vi "ma_SML Averaged Frequency Response.vi"(6 "reset averaging?":bool, 7 "averaging parameters":T1={"averaging type"=enum."no averaging", "averaging settings"={"weighting type"=enum."linear", "weighting settings"={"size"=10.0, "linear weighting mode"=enum."moving average"}}}, 8 "error in (no error)":errorcluster, 9 "spectral info in":T3 {"window" items=["Rectangle"=0, "Hanning"=1, "Hamming"=2, "Blackman-Harris"=3, "Exact Blackman"=4, "Blackman"=5, "Flat Top"=6, "4 Term B-Harris "=7, "7 Term B-Harris"=8, "Low Sidelobe"=9, "Blackman Nuttall"=11, "Triangle"=30, "Bartlett-Hanning"=31, "Bohman"=32, "Parzen"=33, "Welch"=34, "Kaiser"=60, "Dolph-Chebyshev"=61, "Gaussian"=62]}, 10 "FFTspectrum 2":T4 {"spectrum" format="%.2f"; "df" format="%.2f"; "f0" format="%.2f"}, 11 "FFTspectrum 1":T4 {"spectrum" format="%.2f"; "df" format="%.2f"; "f0" format="%.2f"}) -> (0 "error out":errorcluster, 1 "data ready?":bool, 2 "spectral info out":T3 {"window" items=["Rectangle"=0, "Hanning"=1, "Hamming"=2, "Blackman-Harris"=3, "Exact Blackman"=4, "Blackman"=5, "Flat Top"=6, "4 Term B-Harris "=7, "7 Term B-Harris"=8, "Low Sidelobe"=9, "Blackman Nuttall"=11, "Triangle"=30, "Bartlett-Hanning"=31, "Bohman"=32, "Parzen"=33, "Welch"=34, "Kaiser"=60, "Dolph-Chebyshev"=61, "Gaussian"=62]}, 3 "averaged frequency response":T4 {"spectrum" format="%.2f"; "df" format="%.2f"; "f0" format="%.2f"}, 4 "averages sofar":dbl)   [LabVIEW 2020, in "NI_MAPro.lvlib"]
uses:
  NI_MAPro.lvlib
  ma_sml_Spectrum Cluster (complex).ctl
  ma_sml_Spectral Info.ctl
  ma_sml_Averaging Parameters.ctl
  ma_sml_Averaging Settings.ctl
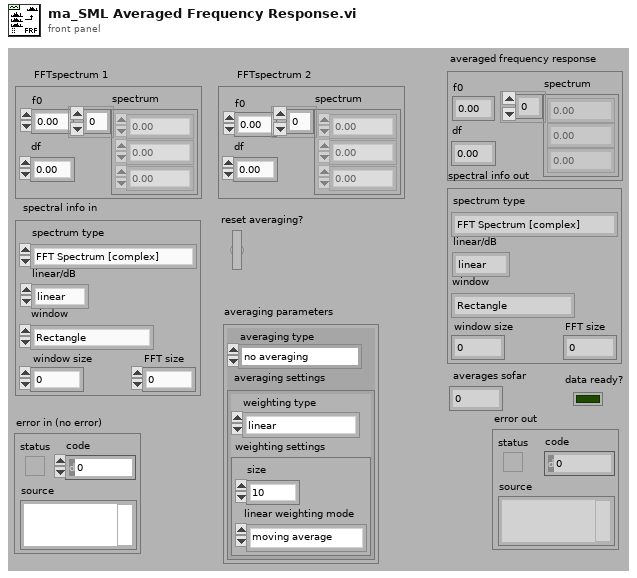
[diagram p1: front panel]
types:
  T1 = typedef "NI_MAPro.lvlib/ma_sml_Averaging Parameters.ctl" = cluster{"averaging type":enum16{"no averaging", "vector averaging", "RMS averaging", "peak hold"}, "averaging settings":T2}
  T2 = typedef "NI_MAPro.lvlib/ma_sml_Averaging Settings.ctl" = cluster{"weighting type":enum16{"linear", "exponential"}, "weighting settings":cluster{"size":dbl, "linear weighting mode":enum16{"one shot", "auto restart one shot", "moving average", "continuous"}}}
  T3 = typedef "NI_MAPro.lvlib/ma_sml_Spectral Info.ctl" = cluster{"spectrum type":enum16{"FFT Spectrum [complex]", "Amplitude [Magnitude]", "Power [Magnitude^2]", "Cross Spectrum [complex]", "Frequency Response [Complex]"}, "linear/dB":enum16{"linear", "dB"}, "window":u16, "window size":i32, "FFT size":i32}
  T4 = typedef "NI_MAPro.lvlib/ma_sml_Spectrum Cluster (complex).ctl" = cluster{"f0":dbl, "df":dbl, "spectrum":cdb[]}
  T5 = enum16{"FFT Spectrum [complex]", "Amplitude [Magnitude]", "Power [Magnitude^2]", "Cross Spectrum [complex]", "Frequency Response [Complex]"}
  T6 = enum16{"no averaging", "vector averaging", "RMS averaging", "peak hold"}
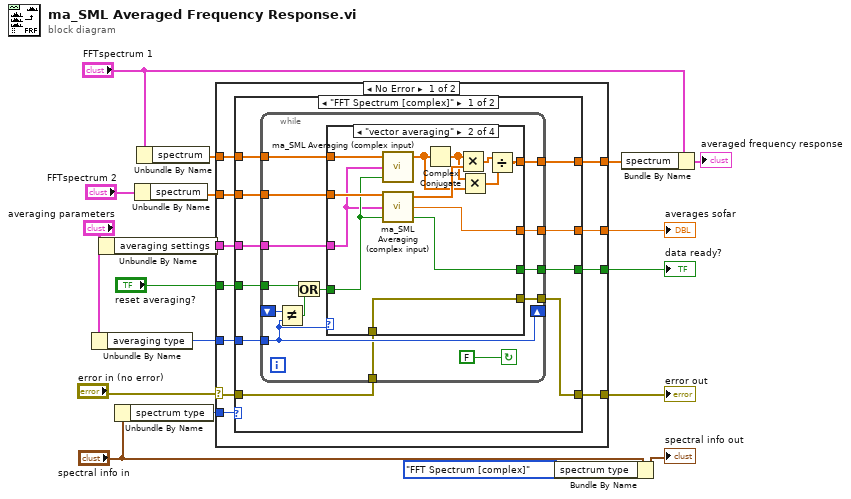
[diagram p0: block diagram]
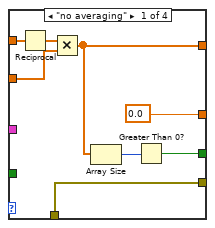
[diagram p2: hidden frame]
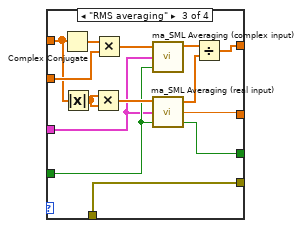
[diagram p3: hidden frame]
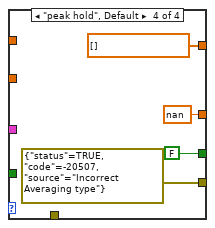
[diagram p4: hidden frame]
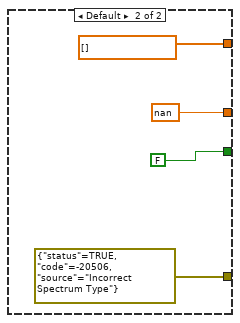
[diagram p5: hidden frame]
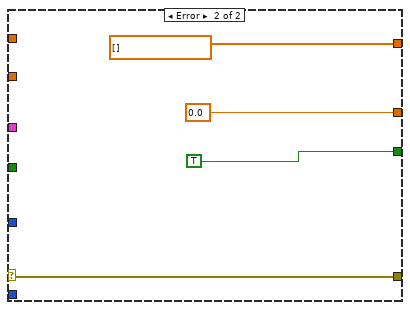
[diagram p6: hidden frame]
diagram:
  n1 = Unbundle By Name("averaging parameters") -> ("averaging type"=w3:T6)
  n2 = Unbundle By Name("averaging parameters") -> ("averaging settings"=w4:T2)
  n3 = Unbundle By Name("spectral info in") -> ("spectrum type"=w7:T5)
  n4 = Unbundle By Name("FFTspectrum 2") -> ("spectrum"=w14:cdb[])
  n5 = Unbundle By Name("FFTspectrum 1") -> ("spectrum"=w13:cdb[])
  n6 = case shown="No Error" "error in (no error)" {
    selector: "error in (no error)" -> [w19 w97]
    tunnel: [w26 TRUE] -> w16
    tunnel: [w24 0.0 ("Averaged So-far")] -> w18
    tunnel: "reset averaging?" -> [w22 _]
    tunnel: w3 -> [w23 _]
    tunnel: [w25 cdb[] [] ("Y")] -> w10
    tunnel: w13 -> [w28 _]
    tunnel: w14 -> [w27 _]
    tunnel: w4 -> [w29 _]
    tunnel: w7 -> [w21 _]
    tunnel: [w20 w97] -> w1
    frame No Error {
      n7 = case shown="\"FFT Spectrum [complex]\"" w21 {
        tunnel: w29 -> [w39 _]
        tunnel: w28 -> [w34 _]
        tunnel: w27 -> [w33 _]
        tunnel: [w32 FALSE] -> w26
        tunnel: [w38 cdb[] []] -> w25
        tunnel: [w37 nan ("Averaged So-far")] -> w24
        tunnel: w23 -> [w36 _]
        tunnel: w22 -> [w35 _]
        tunnel: [w31 errorcluster {"status"=TRUE, "code"=-20506, "source"="Incorrect Spectrum Type"} ("error in (no error)")] -> w20
        tunnel: w19 -> [w30 _]
        frame "FFT Spectrum [complex]" {
          n8 = while {
            tunnel: w30 -> [w40]
            tunnel: [w41] -> w31
            tunnel: w35 -> [w43]
            tunnel: w39 -> [w44]
            shift-left: _ -> [w47]
            shift-right: [w45] -> _
            tunnel: w33 -> [w49]
            tunnel: w34 -> [w50]
            tunnel: [w51] -> w38
            tunnel: w36 -> [w45]
            tunnel: [w52] -> w37
            tunnel: [w53] -> w32
            stop <- FALSE continue-if-true
            n9 = Not Equal?(x=w47, y=w45) -> (x != y?=w46:bool)
            n10 = Or(x=w43, y=w46) -> (x .or. y?=w48:bool)
            n11 = case shown="\"vector averaging\"" w45 {
              tunnel: [w59 w71 w78 FALSE ("Data Ready")] -> w53
              tunnel: [0.0 ("Averaged So-far") w72 w79 nan ("Averaged So-far")] -> w52
              tunnel: w48 -> [_ w73 w77 _]
              tunnel: [w54 w65 w81 cdb[] []] -> w51
              tunnel: w50 -> [w55 w69 w84 _]
              tunnel: w49 -> [w56 w74 w87 _]
              tunnel: w44 -> [_ w68 w76 _]
              tunnel: [w58 w66 w75 errorcluster {"status"=TRUE, "code"=-20507, "source"="Incorrect Averaging type"} ("error out")] -> w41
              tunnel: w40 -> [w58 w66 w75 _]
              frame "no averaging" {
                n12 = Reciprocal(x=w55) -> (1/x=w57:cdb[])
                n13 = Multiply(x=w57, y=w56) -> (x*y=w54:cdb[])
                n14 = Array Size(array=w54) -> (size(s)=w60:i32)
                n15 = Greater Than 0?(x=w60) -> (x > 0?=w59:bool)
              }
              frame "vector averaging" {
                n16 = call "ma_SML Averaging (complex input).vi"("reset?"=w73, "averaging settings"=w68, "x"=w69) -> ("y"=w62:cdb[])  [unwired: 2 out]
                n17 = call "ma_SML Averaging (complex input).vi"("reset?"=w73, "averaging settings"=w68, "x"=w74) -> ("data ready?"=w71:bool, "averaged sofar"=w72:dbl, "y"=w67:cdb[])
                n18 = Complex Conjugate(1:w62) -> (0:w63:cdb[])
                n19 = Multiply(x=w63, y=w67) -> (x*y=w70:cdb[])
                n20 = Multiply(x=w63, y=w62) -> (x*y=w64:cdb[])
                n21 = Divide(x=w70, y=w64) -> (x/y=w65:cdb[])
              }
              frame "RMS averaging" {
                n22 = Complex Conjugate(1:w84) -> (0:w88:cdb[])
                n23 = Absolute Value(x=w84) -> (abs(x)=w82:dbl[])
                n24 = Multiply(x=w82, y=w82) -> (x*y=w83:dbl[])
                n25 = Multiply(x=w88, y=w87) -> (x*y=w86:cdb[])
                n26 = call "ma_SML Averaging (complex input).vi"("reset?"=w77, "averaging settings"=w76, "x"=w86) -> ("y"=w85:cdb[])  [unwired: 2 out]
                n27 = call "ma_SML Averaging (real input).vi"("reset?"=w77, "averaging settings"=w76, "x"=w83) -> ("data ready?"=w78:bool, "averaged sofar"=w79:dbl, "y"=w80:dbl[])
                n28 = Divide(x=w85, y=w80) -> (x/y=w81:cdb[])
              }
              frame "peak hold", Default {
              }
            }
          }
        }
        frame Default {
        }
      }
    }
    frame Error {
    }
  }
  "averages sofar" <- w18
  "data ready?" <- w16
  "error out" <- w1
  n29 = Bundle By Name(cluster="spectral info in", "spectrum type"=T5."FFT Spectrum [complex]") -> (→"spectral info out":T3)
  n30 = Bundle By Name(cluster="FFTspectrum 1", "spectrum"=w10) -> (→"averaged frequency response":T4)
